vi "Silo Mem Test.vi"() -> (1 "return value":i32, 2 "pnTestResult":i32, 3 "Pass?":bool)   [LabVIEW 2015]
doc: "This function will command the DSP to run its Silo memory test.\nPASSED = 1\nFAILED = 0"
uses:
  ScannerDiagDLL.dll
panel:
  out "error out":errorcluster
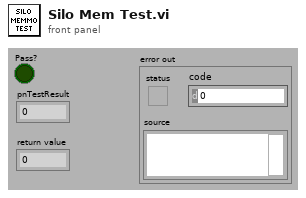
[diagram p1: front panel]
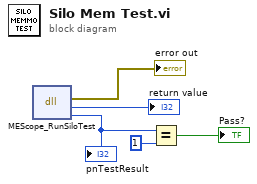
[diagram p0: block diagram]
diagram:
  n1 = dll-call lib="C:/SNAPON/ModisEdge/TabletScope/Test Sequence/Code Modules/DLL/ScannerDiagDLL.dll" fn="MEScope_RunSiloTest"() -> (error out=→"error out":errorcluster, "return type"=→"return value":i32, "*pnTestResult"=w3:i32)  [unwired: 4 in, 1 out]
  "pnTestResult" <- w3
  n2 = Equal?(x=w3, y=1) -> (x = y?=→"Pass?":bool)
